vi "Periodic Tasks.vi"(8 "error in":errorcluster) -> ()   [LabVIEW 2016]
doc: "This VI runs in parallel to other tasks. It can contain as many user-defined periodic loops as you need. These can carry out PID or other sorts of timed response."
uses:
  <vilib>/Rock Robotics/WPI/ThirdParty/CanMotor/TalonSRX/WPI_CANTalonSRX_APIFeedbackSelect.ctl
  <vilib>/Rock Robotics/WPI/Utilities/WPI_GetSetVariantRefNum.vi
  <vilib>/Instr/_visa.llb/VISA Configure Serial Port (Instr).vi
panel:
  out "Positions":i32[](array[numeric])
  out "I2C Out":u8[](array[numeric])
  in  "input string":string
  out "error out":errorcluster
  out "Data Out 3":u8[](array[numeric])
  in  "Numeric":i32
  out "error out 2":errorcluster
  in  "write buffer":string
  out "read buffer":string
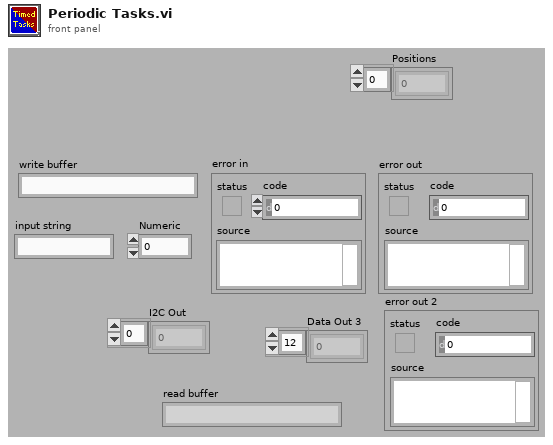
[diagram p1: front panel]
types:
  T1 = typedef "WPI_CANTalonSRX_APIFeedbackSelect.ctl" = enum16{"Digital Quadrature Encoder", "Analog Potentiometer", "Analog Encoder", "Count on Quad-A (Rising-Edge)", "Count on Quad-A (Falling-Edge)", "CTR Magnetic Enc (Absolute)", "CTR Magnetic Enc (Relative)", "Pulse Width"}
  T2 = typedef "WPI_SPIDevRef.ctl" = cluster{"DevStatus":errorcluster, "Handle":i32, "SPI Bus":T3}
  T3 = typedef "spi_bus.ctl" = enum16{"SPI On-Board, CS0", "SPI On-Board, CS1", "SPI On-Board, CS2", "SPI On-Board, CS3", "SPI MXP", "Invalid"}
  T4 = typedef "WPI_I2CDevRef.ctl" = cluster{"DevStatus":errorcluster, "Device Address":u8, "Handle":i32, "I2C Bus":T5}
  T5 = typedef "i2c_bus.ctl" = enum16{"I2C On-Board", "I2C MXP", "Invalid"}
  T6 = typedef "WPI_JoystickDevRef.ctl" = cluster{"Device":T7}
  T7 = typedef "WPI_JoystickDeviceEnum.ctl" = enum16{"USB 0", "USB 1", "USB 2", "USB 3", "USB 4", "USB 5"}
  T8 = typedef "WPI_MotorControlDeviceRef.ctl" = cluster{"DeviceStatus":errorcluster, "Type":T9, "PWM":cluster{"PWM Channel":T10, "DeadBand":T11}, "CAN":cluster{"Device Number":u8, "SetOutput VI Ref":variant, "GetOutput VI Ref":variant, "Enable VI Ref":variant, "Disable VI Ref":variant, "Data":variant}, "Invert":bool}
  T9 = typedef "WPI_MotorControlType.ctl" = enum16{"PWM", "CAN"}
  T10 = typedef "FPGA_DIOPWMChannel.ctl" = enum8{"PWM 0", "PWM 1", "PWM 2", "PWM 3", "PWM 4", "PWM 5", "PWM 6", "PWM 7", "PWM 8", "PWM 9", "PWM MXP 0", "PWM MXP 1", "PWM MXP 2", "PWM MXP 3", "PWM MXP 4", "PWM MXP 5", "PWM MXP 6", "PWM MXP 7", "PWM MXP 8", "PWM MXP 9", "Invalid"}
  T11 = typedef "WPI_PWMDeadband.ctl" = cluster{"Name":string, "maxPositivePwm":i32, "minPositivePwm":i32, "centerPwm":i32, "maxNegativePwm":i32, "minNegativePwm":i32, "angularRange":u16}
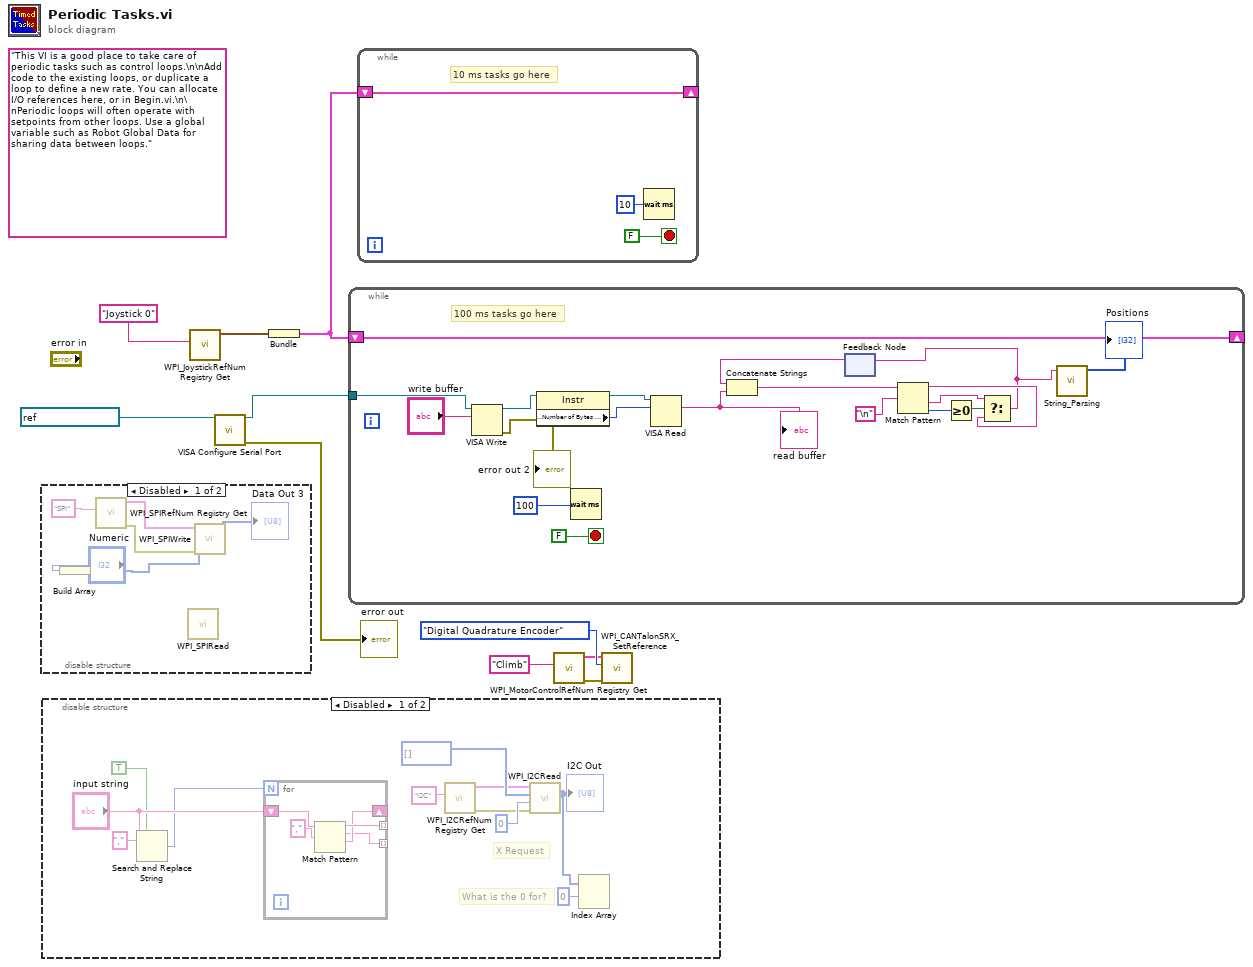
[diagram p0: block diagram]
diagram:
  (unwired) "This VI is a good place to take care of periodic tasks such as control loops.\n\nAdd code to the existing loops, or duplicate a loop to define a new rate. You can allocate I/O references here, or in Begin.vi.\n\nPeriodic loops will often operate with setpoints from other loops. Use a global variable such as Robot Global Data for sharing data between loops."
  n1 = disable-structure shown="Disabled" {
    frame Disabled {
      n2 = Build Array("Numeric") -> (w12:i32[])
      n3 = call <vilib>:"WPI_SPIRefNum Registry Get.vi"("refnum name"="SPI") -> ("error out"=w14:errorcluster, "SPIDevRef"=w15:T2)  [unwired: 9 in]
      n4 = call <vilib>:"WPI_SPIRead.vi"() -> ()  [unwired: 9 in, 3 out]
      n5 = call <vilib>:"WPI_SPIWrite.vi"("error in (no error)"=w14, "Data To Send"=w12, "SPIDevRef"=w15) -> ("Received Data"=→"Data Out 3":u8[])  [unwired: 6 in, 2 out]
    }
    frame Enabled {
    }
  }
  n6 = disable-structure shown="Disabled" {
    frame Disabled {
      # "What is the 0 for?"
      # "X Request"
      n7 = Search and Replace String(replace all?=TRUE ("replace all? (F)"), input string="input string", search string=",") -> (number of replacements=w18:i32)  [unwired: 5 in, 3 out]
      n8 = for {
        N: w18 -> [_]
        tunnel: [w31] -> _ mode=indexing
        shift-right: [w29] -> _
        shift-left: "input string" -> [w30]
        tunnel: [w28] -> _ mode=indexing
        n9 = Match Pattern(string=w30, regular expression=",") -> (before substring=w31:string, match substring=w28:string, after substring=w29:string)  [unwired: 1 in, 1 out]
      }
      n10 = call <vilib>:"WPI_I2CRefNum Registry Get.vi"("refnum name"="I2C") -> ("error out"=w21:errorcluster, "I2CDevRef"=w22:T4)  [unwired: 9 in]
      n11 = call <vilib>:"WPI_I2CRead.vi"("error in (no error)"=w21, "I2CBytesToRead"=u8 0, "I2CRegister"=u8[] [], "I2CDevRef"=w22) -> ("Data Out"=w24:u8[])  [unwired: 5 in, 2 out]
      "I2C Out" <- w24
      n12 = Index Array(array=w24, index #1=0 ("index")) -> ()  [unwired: 1 in, 2 out]
    }
    frame Enabled {
    }
  }
  n13 = call <vilib>:"WPI_JoystickRefNum Registry Get.vi"("refnum name"="Joystick 0") -> ("JoystickDevRef"=w5:T6)  [unwired: 1 in, 9 out]
  n14 = call-poly "VISA Configure Serial Port"("VISA resource name"=refnum<visa-resource-name> "ASRL2::INSTR") -> ("VISA resource name out"=w2:refnum<visa-resource-name>, "error out"=→"error out":errorcluster)  [unwired: 13 in]
  n15 = Bundle("JoystickDevRef"=w5) -> (w4:cluster{"JoystickDevRef":T6})  [unwired: 1 out]
  n16 = while {
    shift-right: [w50] -> _
    shift-left: w4 -> [w50]
    tunnel: w2 -> [w48]
    stop <- FALSE stop-if-true
    # "100 ms tasks go here"
    n17 = VISA Write(VISA resource name=w48, write buffer="write buffer") -> (VISA resource name out=w45:refnum<visa-resource-name>, error out=→"error out 2":errorcluster)  [unwired: 1 in, 1 out]
    n18 = property class="Instr"(reference=w45) -> (reference out=w44:refnum<visa-resource-name>, "Serial Settings:Number of Bytes at Serial Port"=w43:u32)  [unwired: 1 in, 1 out]
    n19 = Wait (ms)(milliseconds to wait=u32 100) -> ()  [unwired: 1 out]
    n20 = VISA Read(VISA resource name=w44, byte count=w43) -> (read buffer=w42:string)  [unwired: 1 in, 3 out]
    "read buffer" <- w42
    n21 = feedback #1() -> (w35:string)  [unwired: 1 in]
    n22 = Concatenate Strings(w35, w42) -> (w41:string)
    n23 = Match Pattern(string=w41, regular expression="\n") -> (before substring=w36:string, after substring=w37:string, offset past match=w39:i32)  [unwired: 1 in, 1 out]
    n24 = Greater Or Equal To 0?(x=w39) -> (x >= 0?=w38:bool)
    n25 = Select(t=w37, s=w38, f=w36) -> (s? t:f=w34:string)
    n26 = feedback-in #1(w34) -> ()
    n27 = call "String_Parsing.vi"("Input"=w34) -> ("Positions"=→"Positions":i32[])  [unwired: 10 in]
  }
  n28 = while {
    shift-right: [w52] -> _
    shift-left: w4 -> [w52]
    stop <- FALSE stop-if-true
    # "10 ms tasks go here"
    n29 = Wait (ms)(milliseconds to wait=u32 10) -> ()  [unwired: 1 out]
  }
  n30 = call <vilib>:"WPI_MotorControlRefNum Registry Get.vi"("refnum name"="Climb") -> ("error out"=w7:errorcluster, "MotorControlDevRef"=w8:T8)  [unwired: 9 in]
  n31 = call <vilib>:"WPI_CANTalonSRX_SetReference.vi"("error in (no error)"=w7, "Feedback Reference"=WPI_CANTalonSRX_APIFeedbackSelect."Digital Quadrature Encoder", "CAN Talon SRX Ref"=w8) -> ()  [unwired: 7 in, 2 out]
